vi "Begin.vi"() -> (0 "error out":errorcluster)   [LabVIEW 2012]
doc: "Called before other user functions, this VI is expected to open initial I/O refnums, load in file data, and do all program initialization. Notice that the <B>error out</B> terminal is simply used for data flow. Wiring it to other structures or subVIs ensures that this VI runs first."
uses:
  <vilib>/Rock Robotics/WPI/DriverStation/WPI_DriverStationRobotMode2.ctl
  <vilib>/Rock Robotics/WPI/Joystick/WPI_JoystickDeviceEnum.ctl
  <vilib>/Rock Robotics/SystemInterfaces/DIO/FPGA_DIOPWMChannel.ctl
  <vilib>/Rock Robotics/SystemInterfaces/DIO/FPGA_DIORelayChannel.ctl
  <vilib>/Rock Robotics/SystemInterfaces/Typedef/FPGA_TypedefDigitalModule.ctl
  Robot Global Data.vi
  <vilib>/Rock Robotics/WPI/MotorControl/WPI_MotorControlOpen Victor.vi
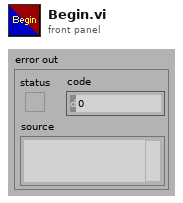
[diagram p1: front panel]
types:
  T1 = typedef "FPGA_DIOPWMChannel.ctl" = enum8{"PWM 1", "PWM 2", "PWM 3", "PWM 4", "PWM 5", "PWM 6", "PWM 7", "PWM 8", "PWM 9", "PWM 10", "Invalid"}
  T2 = typedef "FPGA_TypedefDigitalModule.ctl" = enum16{"Digital Module 1", "Digital Module 2"}
  T3 = typedef "FPGA_DIORelayChannel.ctl" = enum8{"Relay 1", "Relay 2", "Relay 3", "Relay 4", "Relay 5", "Relay 6", "Relay 7", "Relay 8", "Invalid"}
  T4 = typedef "WPI_JoystickDeviceEnum.ctl" = enum16{"USB 1", "USB 2", "USB 3", "USB 4", "Kinect 1", "Kinect 2"}
  T5 = typedef "WPI_DriverStationRobotMode2.ctl" = enum16{"Autonomous Disabled", "Autonomous Enabled", "Teleop Disabled", "Teleop Enabled", "Timeout", "Finish", "Test Disabled", "Test Enabled"}
  T6 = typedef "WPI_JoystickDevRef.ctl" = cluster{"Device":T4}
  T7 = typedef "WPI_MotorControlDeviceRef.ctl" = cluster{"DeviceStatus":errorcluster, "Type":enum16{"PWM", "CAN"}, "PWM":cluster{"Digital Module":T2, "PWM Channel":T1, "DeadBand":T8}, "CAN":cluster{"Device Number":u8, "Control Mode":T9, "Semaphore":T10, "Max Vout":dbl}, "Invert":bool, "TransformRef":T11, "InvTransformRef":T11}
  T8 = typedef "WPI_PWMDeadband.ctl" = cluster{"Name":string, "maxPositivePwm":i32, "minPositivePwm":i32, "centerPwm":i32, "maxNegativePwm":i32, "minNegativePwm":i32, "angularRange":u16}
  T9 = typedef "WPI_CANJaguar_ControlMode.ctl" = enum8{"Percent VBus", "Current", "Speed", "Position", "Voltage"}
  T10 = typedef "Semaphore RefNum" = refnum<k1>
  T11 = typedef "WPI_PWMTransform_ConPane.ctl" = refnum<vi>
  T12 = typedef "WPI_RelayDevRef.ctl" = cluster{"DevStatus":errorcluster, "Relay Channel":T3, "Digital Module":T2, "Relay Direction":T13}
  T13 = typedef "WPI_RelayDirection.ctl" = enum16{"Both directions", "Forward only", "Reverse only"}
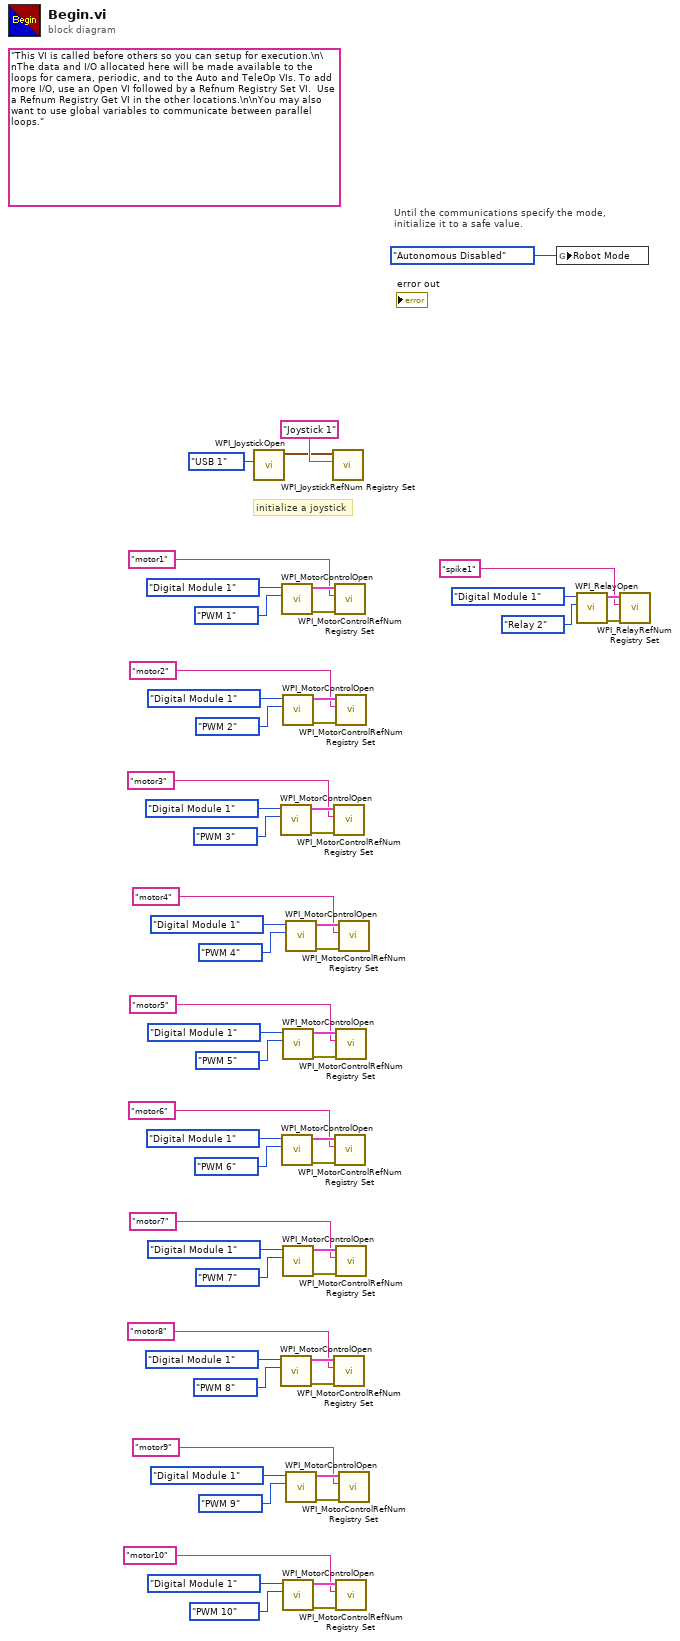
[diagram p0: block diagram]
diagram:
  (unwired) "This VI is called before others so you can setup for execution.\n\nThe data and I/O allocated here will be made available to the loops for camera, periodic, and to the Auto and TeleOp VIs. To add more I/O, use an Open VI followed by a Refnum Registry Set VI.  Use a Refnum Registry Get VI in the other locations.\n\nYou may also want to use global variables to communicate between parallel loops."
  # "initialize a joystick"
  # "Until the communications specify the mode,\ninitialize it to a safe value."
  n1 = call <vilib>:"WPI_JoystickOpen.vi"("JoystickDevice"=WPI_JoystickDeviceEnum."USB 1") -> ("JoystickDevRef"=w57:T6)  [unwired: 10 in]
  n2 = call-poly <vilib>:"WPI_MotorControlOpen.vi"("PWM Channel"=FPGA_DIOPWMChannel."PWM 3", "Digital Module (Module 1)"=FPGA_TypedefDigitalModule."Digital Module 1") -> ("error out"=w44:errorcluster, "MotorControlDeviceRef"=w45:T7)  [unwired: 8 in]
  n3 = call-poly <vilib>:"WPI_MotorControlOpen.vi"("PWM Channel"=FPGA_DIOPWMChannel."PWM 8", "Digital Module (Module 1)"=FPGA_TypedefDigitalModule."Digital Module 1") -> ("error out"=w14:errorcluster, "MotorControlDeviceRef"=w15:T7)  [unwired: 8 in]
  n4 = call-poly <vilib>:"WPI_MotorControlOpen.vi"("PWM Channel"=FPGA_DIOPWMChannel."PWM 1", "Digital Module (Module 1)"=FPGA_TypedefDigitalModule."Digital Module 1") -> ("error out"=w54:errorcluster, "MotorControlDeviceRef"=w55:T7)  [unwired: 8 in]
  n5 = call-poly <vilib>:"WPI_MotorControlOpen.vi"("PWM Channel"=FPGA_DIOPWMChannel."PWM 6", "Digital Module (Module 1)"=FPGA_TypedefDigitalModule."Digital Module 1") -> ("error out"=w24:errorcluster, "MotorControlDeviceRef"=w25:T7)  [unwired: 8 in]
  n6 = call-poly <vilib>:"WPI_MotorControlOpen.vi"("PWM Channel"=FPGA_DIOPWMChannel."PWM 2", "Digital Module (Module 1)"=FPGA_TypedefDigitalModule."Digital Module 1") -> ("error out"=w49:errorcluster, "MotorControlDeviceRef"=w50:T7)  [unwired: 8 in]
  n7 = call-poly <vilib>:"WPI_MotorControlOpen.vi"("PWM Channel"=FPGA_DIOPWMChannel."PWM 5", "Digital Module (Module 1)"=FPGA_TypedefDigitalModule."Digital Module 1") -> ("error out"=w29:errorcluster, "MotorControlDeviceRef"=w30:T7)  [unwired: 8 in]
  n8 = call-poly <vilib>:"WPI_MotorControlOpen.vi"("PWM Channel"=FPGA_DIOPWMChannel."PWM 7", "Digital Module (Module 1)"=FPGA_TypedefDigitalModule."Digital Module 1") -> ("error out"=w19:errorcluster, "MotorControlDeviceRef"=w20:T7)  [unwired: 8 in]
  n9 = call-poly <vilib>:"WPI_MotorControlOpen.vi"("PWM Channel"=FPGA_DIOPWMChannel."PWM 10", "Digital Module (Module 1)"=FPGA_TypedefDigitalModule."Digital Module 1") -> ("error out"=w4:errorcluster, "MotorControlDeviceRef"=w5:T7)  [unwired: 8 in]
  n10 = call-poly <vilib>:"WPI_MotorControlOpen.vi"("PWM Channel"=FPGA_DIOPWMChannel."PWM 4", "Digital Module (Module 1)"=FPGA_TypedefDigitalModule."Digital Module 1") -> ("error out"=w39:errorcluster, "MotorControlDeviceRef"=w40:T7)  [unwired: 8 in]
  n11 = call-poly <vilib>:"WPI_MotorControlOpen.vi"("PWM Channel"=FPGA_DIOPWMChannel."PWM 9", "Digital Module (Module 1)"=FPGA_TypedefDigitalModule."Digital Module 1") -> ("error out"=w9:errorcluster, "MotorControlDeviceRef"=w10:T7)  [unwired: 8 in]
  n12 = call <vilib>:"WPI_JoystickRefNum Registry Set.vi"("refnum name"="Joystick 1", "JoystickDevRef"=w57) -> ()  [unwired: 8 in, 2 out]
  n13 = call <vilib>:"WPI_MotorControlRefNum Registry Set.vi"("error in (no error)"=w44, "refnum name"="motor3", "MotorControlDevRef"=w45) -> ()  [unwired: 7 in, 2 out]
  n14 = call <vilib>:"WPI_MotorControlRefNum Registry Set.vi"("error in (no error)"=w14, "refnum name"="motor8", "MotorControlDevRef"=w15) -> ()  [unwired: 7 in, 2 out]
  n15 = call <vilib>:"WPI_MotorControlRefNum Registry Set.vi"("error in (no error)"=w54, "refnum name"="motor1", "MotorControlDevRef"=w55) -> ()  [unwired: 7 in, 2 out]
  n16 = call <vilib>:"WPI_MotorControlRefNum Registry Set.vi"("error in (no error)"=w24, "refnum name"="motor6", "MotorControlDevRef"=w25) -> ()  [unwired: 7 in, 2 out]
  n17 = call <vilib>:"WPI_MotorControlRefNum Registry Set.vi"("error in (no error)"=w49, "refnum name"="motor2", "MotorControlDevRef"=w50) -> ()  [unwired: 7 in, 2 out]
  n18 = call <vilib>:"WPI_MotorControlRefNum Registry Set.vi"("error in (no error)"=w29, "refnum name"="motor5", "MotorControlDevRef"=w30) -> ()  [unwired: 7 in, 2 out]
  n19 = call <vilib>:"WPI_MotorControlRefNum Registry Set.vi"("error in (no error)"=w19, "refnum name"="motor7", "MotorControlDevRef"=w20) -> ()  [unwired: 7 in, 2 out]
  n20 = call <vilib>:"WPI_MotorControlRefNum Registry Set.vi"("error in (no error)"=w4, "refnum name"="motor10", "MotorControlDevRef"=w5) -> ()  [unwired: 7 in, 2 out]
  n21 = call <vilib>:"WPI_MotorControlRefNum Registry Set.vi"("error in (no error)"=w39, "refnum name"="motor4", "MotorControlDevRef"=w40) -> ()  [unwired: 7 in, 2 out]
  n22 = call <vilib>:"WPI_MotorControlRefNum Registry Set.vi"("error in (no error)"=w9, "refnum name"="motor9", "MotorControlDevRef"=w10) -> ()  [unwired: 7 in, 2 out]
  n23 = global write "Robot Global Data.vi" "Robot Mode"(WPI_DriverStationRobotMode2."Autonomous Disabled" ("Robot Mode")) -> ()
  n24 = call <vilib>:"WPI_RelayOpen.vi"("Relay Channel"=FPGA_DIORelayChannel."Relay 2", "Digital Module (Module 1)"=FPGA_TypedefDigitalModule."Digital Module 1") -> ("error out"=w34:errorcluster, "RelayDevRef"=w35:T12)  [unwired: 8 in]
  n25 = call <vilib>:"WPI_RelayRefNum Registry Set.vi"("error in (no error)"=w34, "refnum name"="spike1", "RelayDevRef"=w35) -> ()  [unwired: 7 in, 2 out]
